vi "U8DigitNumToStr.vi"(11 "U8数组":u8[](array[numeric]) format="%.0x") -> (3 "字符串":string)   [LabVIEW 2012]
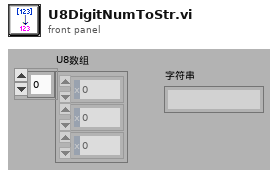
[diagram p1: front panel]
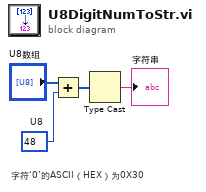
[diagram p0: block diagram]
diagram:
  w3 = u8 48  # U8
  # "字符‘0’的ASCII（HEX）为0X30"
  n1 = Add(x="U8数组", y=w3) -> (x+y=w1:u8[])
  n2 = Type Cast(x=w1) -> (*(type *) &x=→"字符串":string)  [unwired: 1 in]
